vi "TCP Initialization loop.vi"(11 "TCP Port Listen List":u16[](array[numeric])) -> (2 "Array out":errorcluster[](array[cluster]), 3 "output cluster":T1)   [LabVIEW 2016]
uses:
  TCP Port Control.ctl
panel:
  in  "TCP Network Connection in":refnum<k5>
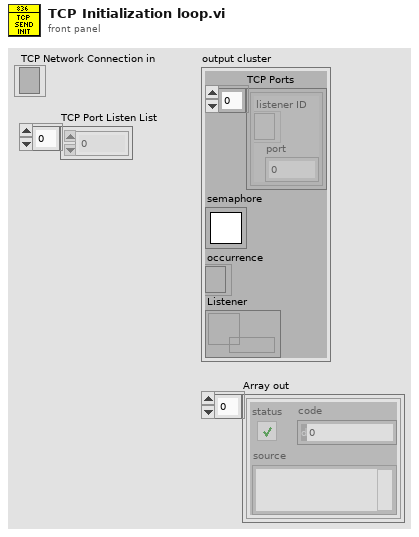
[diagram p1: front panel]
types:
  T1 = typedef "TCP Port Control.ctl" = cluster{"TCP Ports":cluster{"listener ID":refnum<k5>, "port":u16}[], "semaphore":T2, "occurrence":refnum<k4>, "Listener":refnum<data-value>}
  T2 = typedef "Semaphore RefNum" = refnum<k1>
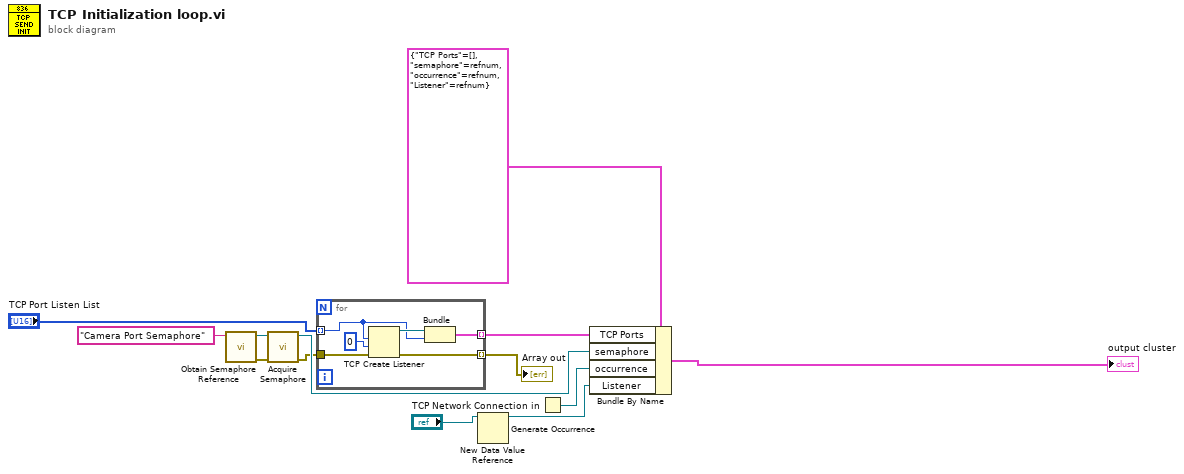
[diagram p0: block diagram]
diagram:
  n1 = call <vilib>:"Obtain Semaphore Reference.vi"("name (unnamed)"="Camera Port Semaphore") -> ("error out"=w4:errorcluster, "semaphore"=w5:T2)  [unwired: 4 in, 1 out]
  n2 = call <vilib>:"Acquire Semaphore.vi"("error in (no error)"=w4, "semaphore"=w5) -> ("error out"=w8:errorcluster, "semaphore out"=w11:T2)  [unwired: 3 in, 1 out]
  n3 = for {
    tunnel: "TCP Port Listen List" -> [w16] mode=indexing
    tunnel: [w15] -> w10 mode=indexing
    tunnel: [w19] -> w7 mode=indexing
    tunnel: w8 -> [w14]
    n4 = TCP Create Listener(8:w14, 9:0 ("timeout ms (25000)"), 10:w16) -> (0:w19:errorcluster, 3:w17:refnum<k5>)  [unwired: 2 in, 1 out]
    n5 = Bundle("listener ID"=w17, "port"=w16) -> (w15:cluster{"listener ID":refnum<k5>, "port":u16})  [unwired: 1 in]
  }
  "Array out" <- w7
  n6 = New Data Value Reference(data value="TCP Network Connection in") -> (data value reference=w13:refnum<data-value>)  [unwired: 1 in, 1 out]
  n7 = Generate Occurrence() -> (w12:refnum<k4>)
  n8 = Bundle By Name(cluster=T1 {"TCP Ports"=[], "semaphore"=refnum, "occurrence"=refnum, "Listener"=refnum} ("output cluster"), "TCP Ports"=w10, "semaphore"=w11, "occurrence"=w12, "Listener"=w13) -> (→"output cluster":T1)
